vi "equal_example.vi"() -> ()   [LabVIEW 2010]
uses:
  <vilib>/AddOns/Modulation/Analog/controls/Complex Data Waveform.ctl
  <vilib>/addons/Modulation/Digital/Impairments/Fading Profiles/MT Rayleigh Fading Profile (Gans).vi
  <vilib>/addons/Modulation/Digital/Impairments/MT Apply Flat Fading Profile.vi
  <vilib>/addons/Adaptive Filters/Create/AFT Create FIR LMS (Complex).vi
  <vilib>/addons/Adaptive Filters/Processing/AFT Filter Signal and Update Coefficients (Complex, Array).vi
  <vilib>/addons/Adaptive Filters/Analysis/AFT Get Coefficients (FIR, Complex).vi
  <vilib>/measure/NI_MABase.lvlib
  <vilib>/addons/Adaptive Filters/NI_AdaptiveFilter.lvlib
  <vilib>/addons/Modulation/niDMT.lvlib
  <vilib>/addons/Modulation/niAMT.lvlib
  <vilib>/Analysis/NI_AALBase.lvlib
  <vilib>/Analysis/3filter.llb/IIR Filter (CDB).vi
panel:
  out "IIR_real 2":dbl[](graph)
  out "IIR_imag 2":dbl[](graph)
  out "contain_real":dbl[](graph)
  out "contain_imag":dbl[](graph)
  out "ADSP_real":dbl[](graph)
  out "ADSP_imag":dbl[](graph)
  out "error":dbl[](graph)
  # "基于LMS算法的信道均衡范例"
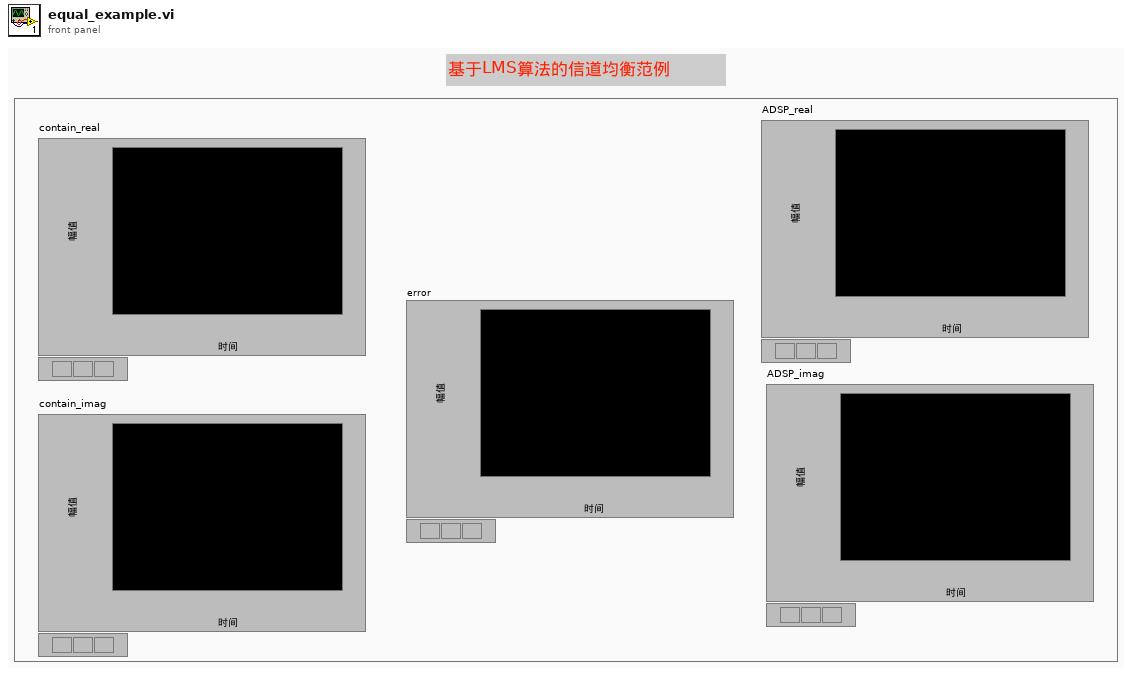
[diagram p1: front panel]
types:
  T1 = enum16{"Sine Wave", "Triangle Wave", "Square Wave", "Sawtooth Wave"}
  T2 = typedef "niAMT.lvlib/Complex Data Waveform.ctl" = cluster{"t0":dbl, "dt":dbl, "Y":cdb[]}
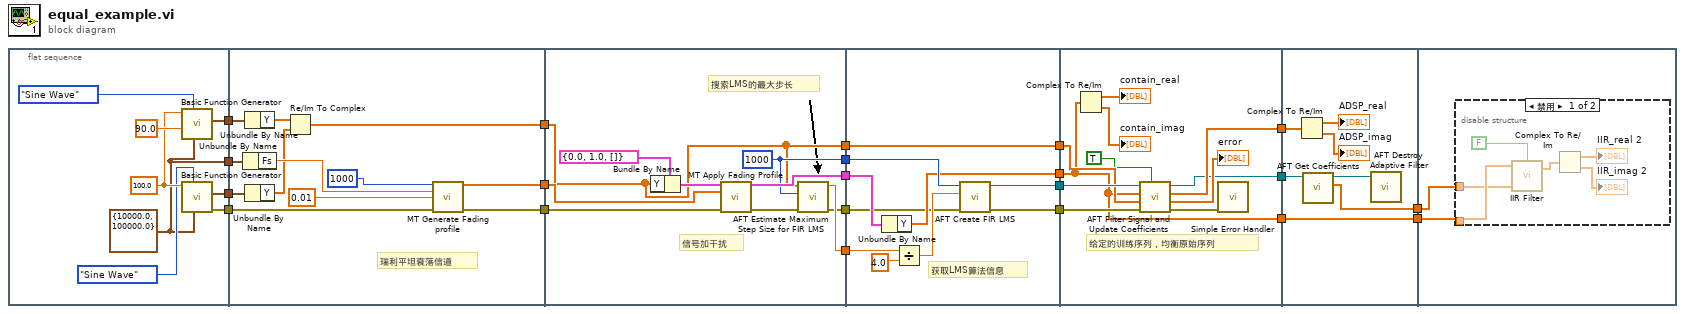
[diagram p0: block diagram]
diagram:
  n1 = flat-sequence {
    tunnel: [w25] -> w21
    tunnel: [w24] -> w18
    tunnel: [w23] -> w17
    tunnel: [w22] -> w16
    tunnel: w21 -> [w38]
    tunnel: [w37] -> w20
    tunnel: [w36] -> w19
    tunnel: w18 -> [w35]
    tunnel: w17 -> [w32]
    tunnel: w16 -> [w31]
    tunnel: [w30] -> w15
    tunnel: w20 -> [w51]
    tunnel: w19 -> [w50]
    tunnel: w15 -> [w43]
    tunnel: [w47] -> w14
    tunnel: [w45] -> w13
    tunnel: [w44] -> w12
    tunnel: [w43] -> w8
    tunnel: [w42] -> w7
    tunnel: w14 -> [w61]
    tunnel: w13 -> [w60]
    tunnel: w12 -> [w58]
    tunnel: [w56] -> w11
    tunnel: [w55] -> w10
    tunnel: [w54] -> w9
    tunnel: w8 -> [w54]
    tunnel: w7 -> [w53]
    tunnel: [w52] -> w6
    tunnel: w11 -> [w72]
    tunnel: w10 -> [w62]
    tunnel: w9 -> [w71]
    tunnel: w6 -> [w70]
    tunnel: [w68] -> w5
    tunnel: [w63] -> w4
    tunnel: [w62] -> w2
    tunnel: w5 -> [w77]
    tunnel: w4 -> [w76]
    tunnel: [w74] -> w3
    tunnel: w2 -> [w74]
    tunnel: [w73] -> w1
    tunnel: w3 -> [w81]
    tunnel: w1 -> [w80]
    frame #0 {
      w25 = cluster{"Fs":dbl, "#s":dbl} {"Fs"=10000.0, "#s"=100000.0} ("sampling info")
      w27 = 100.0 ("frequency")
      n2 = call <vilib>:"Basic Function Generator.vi"("sampling info"=w25, "signal type"=T1."Sine Wave", "phase"=90.0, "frequency"=w27) -> ("signal out"=w23:waveform(dbl))  [unwired: 5 in, 2 out]
      n3 = call <vilib>:"Basic Function Generator.vi"("sampling info"=w25, "signal type"=T1."Sine Wave", "frequency"=w27) -> ("error out"=w24:errorcluster, "signal out"=w22:waveform(dbl))  [unwired: 6 in, 1 out]
    }
    frame #1 {
      # "瑞利平坦衰落信道"
      n4 = Unbundle By Name(w38) -> ("Fs"=w40:dbl)
      n5 = Unbundle By Name(w32) -> ("Y"=w33:dbl[])
      n6 = Unbundle By Name(w31) -> ("Y"=w34:dbl[])
      n7 = Re/Im To Complex(1:w34, 2:w33) -> (0:w30:cdb[])
      n8 = call-poly <vilib>:"MT Generate Fading profile.vi"("profile length (samples)"=1000, "sampling frequency (Hz)"=w40, "doppler spread (Hz)"=0.01, "error in (no error)"=w35) -> ("fading profile"=w37:cdb[], "error out"=w36:errorcluster)  [unwired: 9 in, 1 out]
    }
    frame #2 {
      w45 = 1000 ("filter length")
      # "信号加干扰"
      # "搜索LMS的最大步长"
      n9 = Bundle By Name(cluster=T2 {"t0"=0.0, "dt"=1.0, "Y"=[]} ("input complex waveform"), "Y"=w43) -> (w48:T2)
      n10 = call-poly <vilib>:"MT Apply Fading Profile.vi"("input complex waveform"=w48, "fading profile"=w51, "error in (no error)"=w50) -> ("output complex waveform"=w47:T2, "error out"=w46:errorcluster)  [unwired: 11 in]
      n11 = call <vilib>:"AFT Estimate Maximum Step Size for FIR LMS.vi"("error in (no error)"=w46, "filter length"=w45, "x(n)"=w43) -> ("error out"=w42:errorcluster, "maximum step size"=w44:dbl)  [unwired: 7 in]
    }
    frame #3 {
      # "获取LMS算法信息"
      n12 = Unbundle By Name(w61) -> ("Y"=w55:cdb[])
      n13 = Divide(x=w58, y=4.0) -> (x/y=w57:dbl)
      n14 = call-poly <vilib>:"AFT Create FIR LMS.vi"("error in (no error)"=w53, "step size"=w57, "filter length"=w60) -> ("error out"=w52:errorcluster, "adaptive filter out"=w56:refnum<k20>)  [unwired: 7 in]
    }
    frame #4 {
      # "给定的训练序列，均衡原始序列"
      n15 = Complex To Re/Im(x + iy=w62) -> (x=→"contain_real":dbl[], y=→"contain_imag":dbl[])
      n16 = call-poly <vilib>:"AFT Filter Signal and Update Coefficients.vi"("reset? (F)"=TRUE, "error in (no error)"=w70, "d(n)"=w71, "x(n)"=w62, "adaptive filter in"=w72) -> ("error out"=w66:errorcluster, "e(n)"=→"error":cdb[], "y(n)"=w68:cdb[], "adaptive filter out"=w63:refnum<k20>)  [unwired: 3 in]
      n17 = call <vilib>:"Simple Error Handler.vi"("error in (no error)"=w66) -> ()  [unwired: 4 in, 5 out]
    }
    frame #5 {
      n18 = Complex To Re/Im(x + iy=w77) -> (x=→"ADSP_real":dbl[], y=→"ADSP_imag":dbl[])
      n19 = call-poly <vilib>:"AFT Get Coefficients.vi"("adaptive filter in"=w76) -> ("coefficients"=w73:cdb[], "adaptive filter out"=w75:refnum<k20>)  [unwired: 8 in, 1 out]
      n20 = call <vilib>:"AFT Destroy Adaptive Filter.vi"("adaptive filter in"=w75) -> ()  [unwired: 10 in, 1 out]
    }
    frame #6 {
      n21 = disable-structure shown="禁用" {
        disable-tunnel: w81 -> [w86 _]
        disable-tunnel: w80 -> [w85 _]
        frame Disabled {
          n22 = call-poly <vilib>:"IIR Filter.vi"("init/cont (init:F)"=FALSE, "Forward Coefficients"=w85, "X"=w86) -> ("Filtered X"=w82:cdb[])  [unwired: 1 in, 1 out]
          n23 = Complex To Re/Im(x + iy=w82) -> (x=→"IIR_real 2":dbl[], y=→"IIR_imag 2":dbl[])
        }
        frame Enabled {
        }
      }
    }
  }
